vi "Puff_using_Arduino.vi"(2 "Time to hold source ON (microseconds)":u32=100000 format="%.0g", 3 "Time to hold source OFF (microseconds)":u32=1000000 format="%.0g", 4 "Number of cycles":u16=5) -> (0 "error out":errorcluster, 1 "Completed cycles":u16=5)   [LabVIEW 2012]
uses:
  Arduino_comms_Global.vi
panel:
  out "bytes sent":u32=12
  out "write buffer":string
  # "Paul Nathan, 18/06/2013"
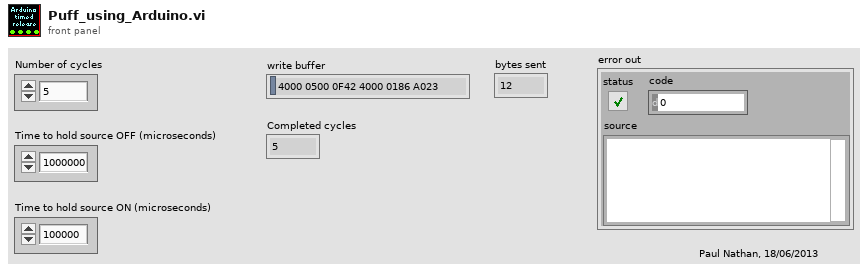
[diagram p1: front panel]
types:
  T1 = typedef "Arduino_comm_params.ctl" = cluster{"VISA resource name":refnum<visa-resource-name>, "byte count":u32, "flow control (0:none)":u16, "stop bits (10: 1 bit)":u16, "parity (0:none)":enum16{"None", "Odd", "Even", "Mark", "Space"}, "data bits (8)":u16, "termination char ":u8, "Enable Termination\nChar":bool, "baud rate (bps)":u32, "timeout (ms)":u32, "Locked":bool}
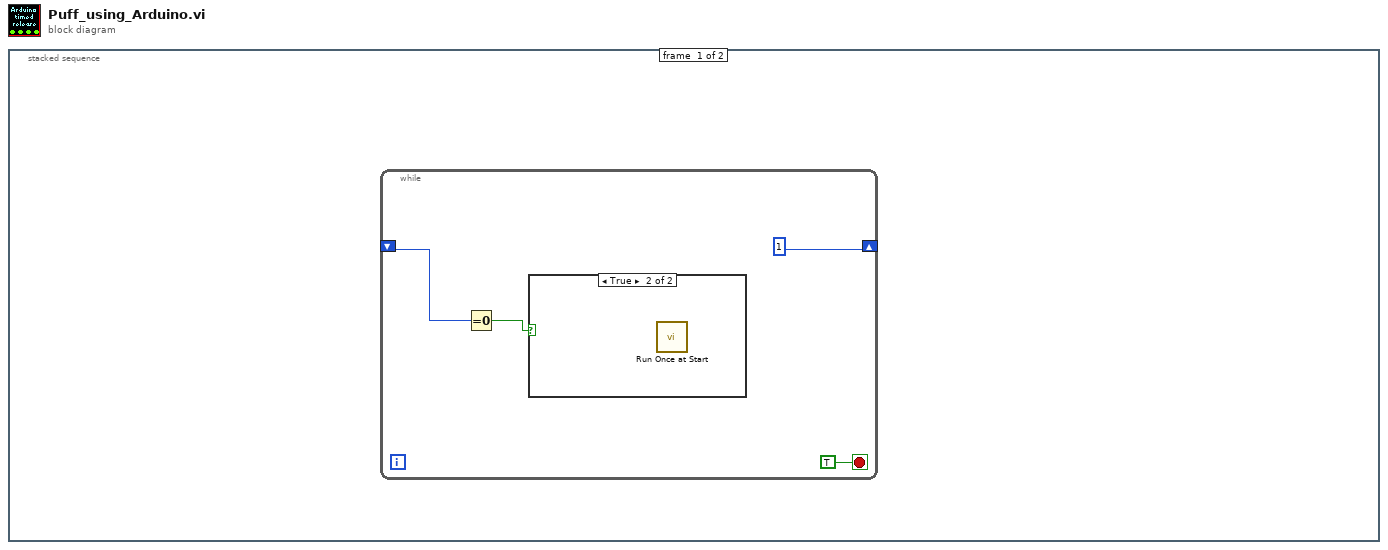
[diagram p0: block diagram]
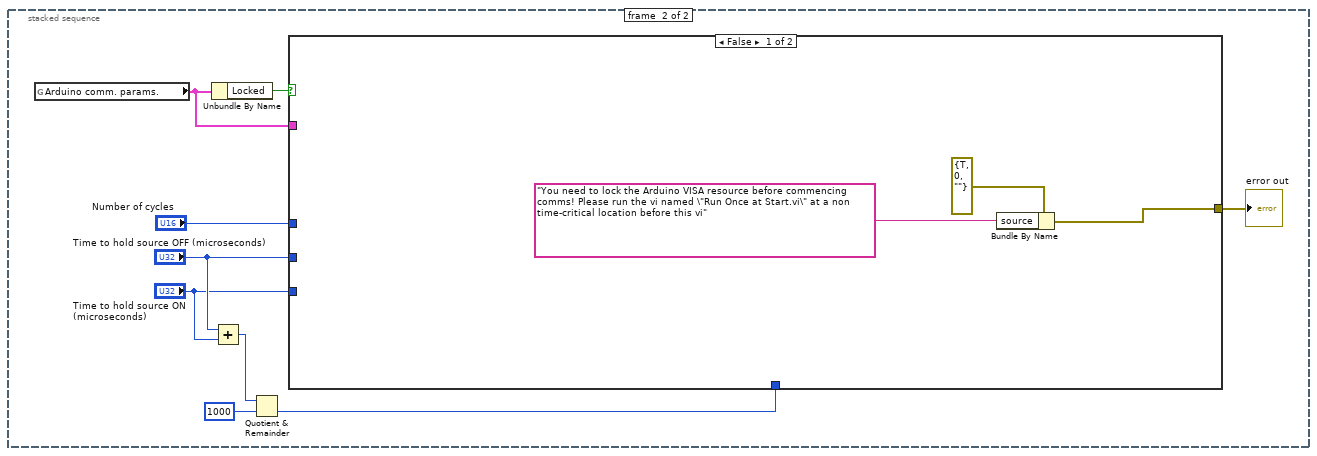
[diagram p3: hidden frame]
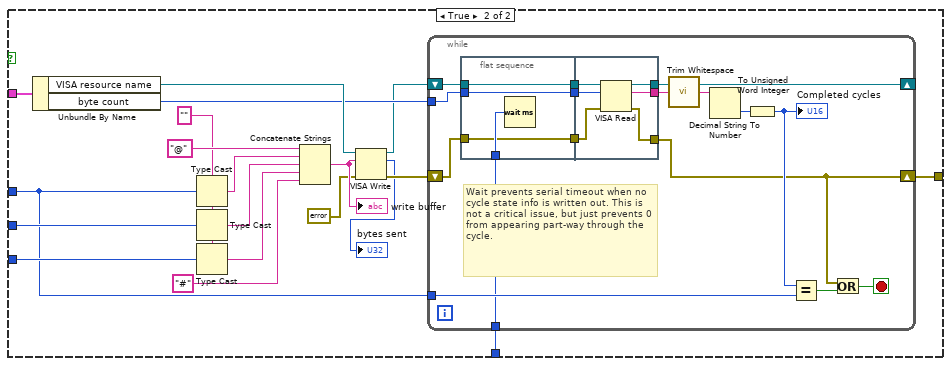
[diagram p4: hidden frame]
diagram:
  n1 = stacked-sequence {
    frame #0 {
      n2 = while {
        shift-right: [1] -> _
        shift-left: _ -> [w4]
        stop <- TRUE stop-if-true
        n3 = Equal To 0?(x=w4) -> (x = 0?=w3:bool)
        n4 = case shown="True" w3 {
          frame False {
          }
          frame True {
            n5 = call "Run Once at Start.vi"() -> ()  [unwired: 1 in]
          }
        }
      }
    }
    frame #1 {
      n6 = global read "Arduino_comms_Global.vi" "Arduino comm. params."() -> (w12:T1)
      n7 = Unbundle By Name(w12) -> ("Locked"=w13:bool)
      n8 = Add(x="Time to hold source OFF (microseconds)", y="Time to hold source ON (microseconds)") -> (x+y=w7:u32)
      n9 = Quotient & Remainder(x=w7, y=u32 1000) -> (floor(x/y)=w5:u32)  [unwired: 1 out]
      n10 = case shown="False" w13 {
        tunnel: w12 -> [_ w33]
        tunnel: "Number of cycles" -> [_ w21]
        tunnel: "Time to hold source OFF (microseconds)" -> [_ w31]
        tunnel: "Time to hold source ON (microseconds)" -> [_ w30]
        tunnel: [w14 w23] -> w10
        tunnel: w5 -> [_ w17]
        frame False {
          n11 = Bundle By Name(cluster=errorcluster {"status"=TRUE, "code"=0, "source"=""} ("error out"), "source"="You need to lock the Arduino VISA resource before commencing comms! Please run the vi named \"Run Once at Start.vi\" at a non time-critical location before this vi") -> (w14:errorcluster)
        }
        frame True {
          w32 = ""
          n12 = Unbundle By Name(w33) -> ("VISA resource name"=w26:refnum<visa-resource-name>, "byte count"=w25:u32)
          n13 = Type Cast(type=w32, x=w21) -> (*(type *) &x=w29:string)
          n14 = Type Cast(type=w32, x=w31) -> (*(type *) &x=w28:string)
          n15 = Type Cast(type=w32, x=w30) -> (*(type *) &x=w27:string)
          n16 = Concatenate Strings("@", w29, w28, w27, "#") -> (w34:string)
          "write buffer" <- w34
          n17 = VISA Write(VISA resource name=w26, write buffer=w34, error in (no error)=errorcluster {"status"=FALSE, "code"=0, "source"=""}) -> (VISA resource name out=w20:refnum<visa-resource-name>, return count=→"bytes sent":u32, error out=w24:errorcluster)
          n18 = while {
            tunnel: w25 -> [w50]
            shift-right: [w38] -> w23
            shift-left: w24 -> [w40]
            shift-right: [w49] -> _
            shift-left: w20 -> [w51]
            tunnel: w21 -> [w47]
            tunnel: w17 -> [w41]
            stop <- w36 stop-if-true
            # "Wait prevents serial timeout when no cycle state info is written out. This is not a critical issue, but just prevents 0 from appearing part-way through the cycle."
            n19 = flat-sequence {
              tunnel: w50 -> [w54]
              tunnel: w51 -> [w55]
              tunnel: [w55] -> w43
              tunnel: [w54] -> w42
              tunnel: w41 -> [w53]
              tunnel: w40 -> [w52]
              tunnel: [w52] -> w39
              tunnel: [w59] -> w49
              tunnel: [w58] -> w45
              tunnel: w43 -> [w61]
              tunnel: w42 -> [w60]
              tunnel: w39 -> [w57]
              tunnel: [w56] -> w38
              frame #0 {
                n20 = Wait (ms)(milliseconds to wait=w53) -> ()  [unwired: 1 out]
              }
              frame #1 {
                n21 = VISA Read(VISA resource name=w61, byte count=w60, error in (no error)=w57) -> (VISA resource name out=w59:refnum<visa-resource-name>, read buffer=w58:string, error out=w56:errorcluster)  [unwired: 1 out]
              }
            }
            n22 = call <vilib>:"Trim Whitespace.vi"("string"=w45) -> ("trimmed string"=w44:string)  [unwired: 1 in]
            n23 = Decimal String To Number(string=w44) -> (number=w48:i32)  [unwired: 2 in, 1 out]
            n24 = To Unsigned Word Integer(number=w48) -> (unsigned 16bit integer=w46:u16)
            "Completed cycles" <- w46
            n25 = Equal?(x=w46, y=w47) -> (x = y?=w37:bool)
            n26 = Or(x=w38, y=w37) -> (x .or. y?=w36:bool)
          }
        }
      }
      "error out" <- w10
    }
  }
